vi "Convert Number to String and Pad with Zeroes.vi"(9 "Minimum Width":i16=1 min=1, 11 "Number":i32) -> (3 "Number in string representation (padded with zeroes)":string)   [LabVIEW 2013]
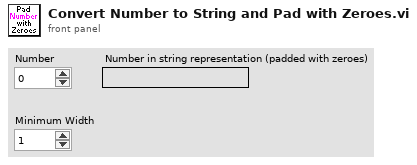
[diagram p1: front panel]
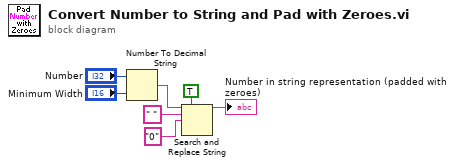
[diagram p0: block diagram]
diagram:
  n1 = Number To Decimal String(number="Number", width (-)="Minimum Width") -> (decimal integer string=w4:string)
  n2 = Search and Replace String(replace all?=TRUE ("replace all? (F)"), input string=w4, search string=" ", replace string="0" ("replace string (\"\")")) -> (result string=→"Number in string representation (padded with zeroes)":string)  [unwired: 4 in, 3 out]
